vi "test _turtur.vi"   [LabVIEW 2015]
uses:
  C:/Users/Andrei/Desktop/work/NI/DLL_ALGO/Debug/DLL_ALGO.dll
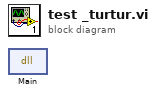
[diagram p0: block diagram]
diagram:
  n1 = dll-call lib="C:/Users/Andrei/Desktop/work/NI/DLL_ALGO/Debug/DLL_ALGO.dll" fn="Main"() -> ()  [unwired: 4 in, 2 out]
